vi "SetMenuPosition.vi"(8 "error in (no error)":errorcluster, 10 "Horizontal":i32, 11 "Vertical":i32) -> (0 "error out":errorcluster)   [LabVIEW 2015]
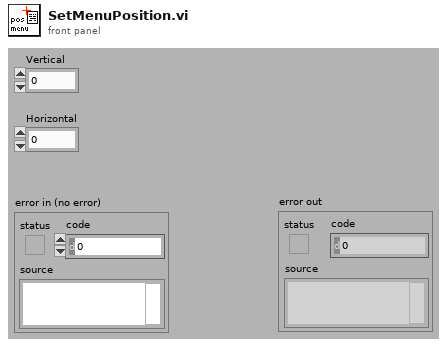
[diagram p1: front panel]
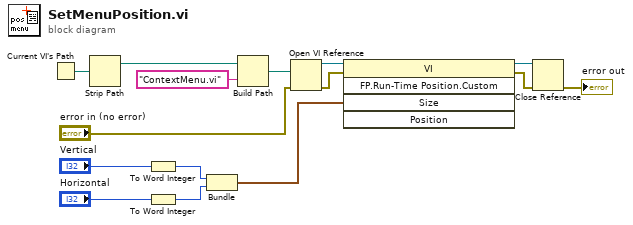
[diagram p0: block diagram]
diagram:
  n1 = Current VI's Path() -> (path=w14:path)
  n2 = Strip Path(path=w14) -> (stripped path=w13:path)  [unwired: 1 out]
  n3 = To Word Integer(number="Vertical") -> (16bit integer=w6:i16)
  n4 = To Word Integer(number="Horizontal") -> (16bit integer=w7:i16)
  n5 = Bundle(w6, w7) -> (w5:cluster{i16, i16})  [unwired: 1 out]
  n6 = Build Path(base path=w13, name or relative path="ContextMenu.vi") -> (appended path=w11:path)
  n7 = Open VI Reference(vi path=w11, error in (no error)="error in (no error)") -> (vi reference=w15:refnum<vi>, error out=w10:errorcluster)  [unwired: 4 out]
  n8 = invoke class="VI" method="FP.Run-Time Position.Custom"(reference=w15, error in=w10, "Size"=w5) -> (reference out=w4:refnum<vi>, error out=w3:errorcluster)  [unwired: 2 in, 3 out]
  n9 = Close Reference(reference=w4, error in (no error)=w3) -> (error out=→"error out":errorcluster)
